vi "Set-Point Experiment Bundle.vi"() -> (0 "Input Channels":string, 1 "Output Channels":string, 2 "Output Waveforms":waveform(dbl)[](array[waveform]))   [LabVIEW 2013]
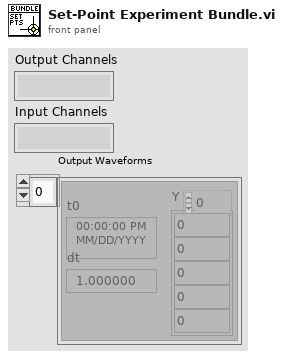
[diagram p1: front panel]
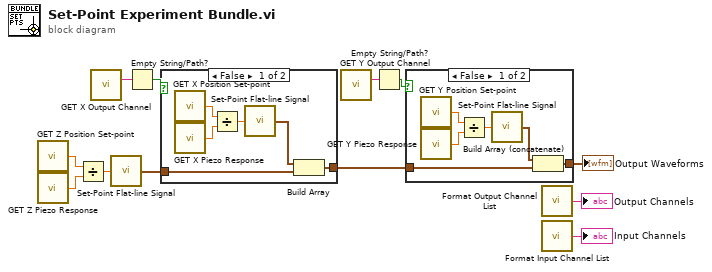
[diagram p0: block diagram]
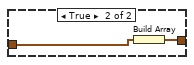
[diagram p3: hidden frame]
diagram:
  n1 = call "GET Z Position Set-point.vi"() -> ("Z Position Set-point"=w6:dbl)
  n2 = call "GET Z Piezo Response.vi"() -> ("Z Piezo Response"=w5:dbl)
  n3 = Divide(x=w6, y=w5) -> (x/y=w4:dbl)
  n4 = call "GET X Output Channel.vi"() -> ("X Output Channel"=w8:string)
  n5 = call "Set-Point Flat-line Signal.vi"("Flatline Offset"=w4) -> ("Flatline Signal"=w3:waveform(dbl))
  n6 = Empty String/Path?(string/path=w8) -> (empty?=w7:bool)
  n7 = case shown="False" w7 {
    tunnel: w3 -> [w15 w19]
    tunnel: [w13 w20] -> w2
    frame False {
      n8 = call "GET X Position Set-point.vi"() -> ("X Position Set-point"=w17:dbl)
      n9 = call "GET X Piezo Response.vi"() -> ("X Piezo Response"=w18:dbl)
      n10 = Divide(x=w17, y=w18) -> (x/y=w16:dbl)
      n11 = call "Set-Point Flat-line Signal.vi"("Flatline Offset"=w16) -> ("Flatline Signal"=w14:waveform(dbl))
      n12 = Build Array(w14, w15) -> (w13:waveform(dbl)[])
    }
    frame True {
      n13 = Build Array(w19) -> (w20:waveform(dbl)[])
    }
  }
  n14 = call "GET Y Output Channel.vi"() -> ("Y Output Channel"=w10:string)
  n15 = Empty String/Path?(string/path=w10) -> (empty?=w9:bool)
  n16 = case shown="False" w9 {
    tunnel: w2 -> [w23 w27]
    tunnel: [w21 w27] -> w1
    frame False {
      n17 = call "GET Y Position Set-point.vi"() -> ("Y Position Set-point"=w25:dbl)
      n18 = call "GET Y Piezo Response.vi"() -> ("Y Piezo Response"=w26:dbl)
      n19 = Divide(x=w25, y=w26) -> (x/y=w24:dbl)
      n20 = call "Set-Point Flat-line Signal.vi"("Flatline Offset"=w24) -> ("Flatline Signal"=w22:waveform(dbl))
      n21 = Build Array (concatenate)(w22, w23) -> (w21:waveform(dbl)[])
    }
    frame True {
    }
  }
  "Output Waveforms" <- w1
  n22 = call "Format Output Channel List.vi"() -> ("Output Channels"=→"Output Channels":string)
  n23 = call "Format Input Channel List.vi"() -> ("Input Channels"=→"Input Channels":string)
